vi "Fortsetzen Reset.vi"(10 "FORTSETZEN":T1, 11 "Referenz Boolesch (Eingang)":refnum<vi>) -> ()   [LabVIEW 2020, in "Linearisierung v2.lvlib" / "SpanEinstellungen.lvlib"]
uses:
  SpanEinstellungen.lvlib
  Visualisierungs Elemente/Button.ctl
  Aktion FGV Stoerungen sammeln und auswerten.ctl
  Linearisierung v2.lvlib
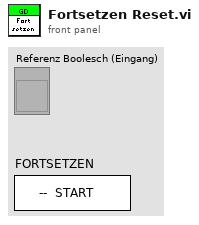
[diagram p1: front panel]
types:
  T1 = typedef "Button.ctl" = bool
  T2 = typedef "Linearisierung v2.lvlib/Aktion FGV Stoerungen sammeln und auswerten.ctl" = enum16{"init", "lesen", "error", "prüfen", "reset error", "abbrechen", "fortsetzen", "neustart", "Bedientasten reset"}
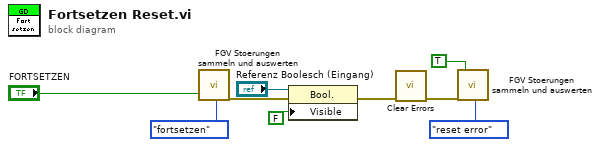
[diagram p0: block diagram]
diagram:
  n1 = call "FGV Stoerungen sammeln und auswerten.vi"("Fortsetzen"="FORTSETZEN", "Aktion"=Aktion_FGV_Stoerungen_sammeln_und_auswerten."fortsetzen") -> ("error out"=w7:errorcluster)  [unwired: 11 in, 6 out]
  n2 = property on="Eigenschaftsknoten" class="Bool."(reference="Referenz Boolesch (Eingang)", error in=w7, "Visible"=FALSE ("Sichtbar")) -> (error out=w5:errorcluster)  [unwired: 1 out]
  n3 = call <vilib>:"Clear Errors.vi"("error in (no error)"=w5) -> ("error out"=w9:errorcluster)  [unwired: 5 in, 1 out]
  n4 = call "FGV Stoerungen sammeln und auswerten.vi"("error in (no error)"=w9, "keep Errors for AutoSPAN"=TRUE, "Aktion"=Aktion_FGV_Stoerungen_sammeln_und_auswerten."reset error") -> ()  [unwired: 10 in, 7 out]
